vi "httpClient.vi"(8 "error in":errorcluster, 10 "data":string, 11 "URI":string) -> (0 "error out":errorcluster, 2 "code create":bool, 3 "HTTP Response Code":i32)   [LabVIEW 2015]
uses:
  <vilib>/httpClient/LabVIEWHTTPClient.lvlib
  <vilib>/Easy HTTP Client/HTTP Header.ctl
panel:
  out "headers":T1[](array[typedef])
  out "body":string
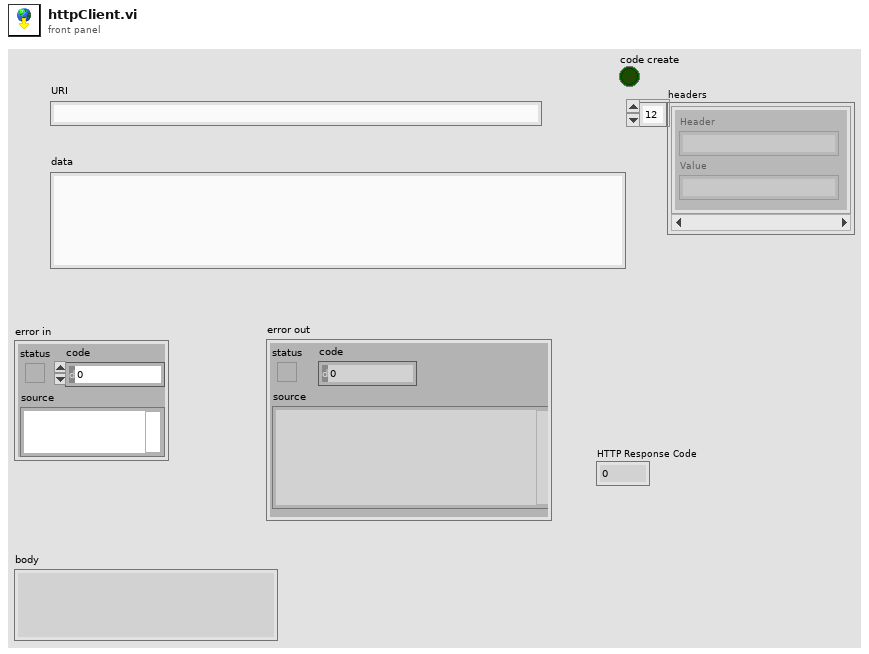
[diagram p1: front panel]
types:
  T1 = typedef "Easy HTTP.lvlib/HTTP Header.ctl" = cluster{"Header":string, "Value":string}
  T2 = typedef "LabVIEWHTTPClient.lvlib/ClientHandle.ctl" = refnum<k1>
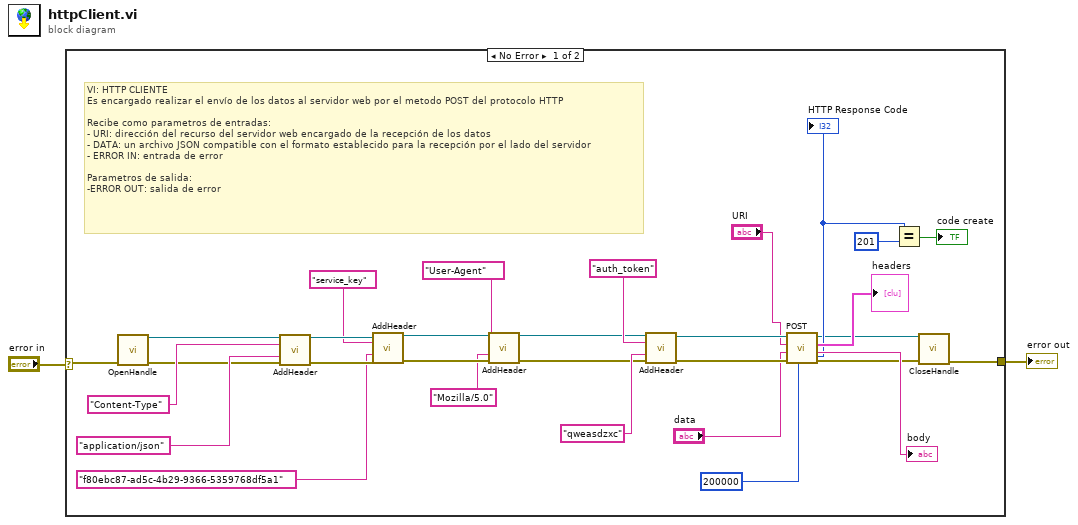
[diagram p0: block diagram]
diagram:
  n1 = case shown="No Error" "error in" {
    selector: "error in" -> [w6 w33]
    tunnel: [w4 w33] -> w1
    frame No Error {
      # "VI: HTTP CLIENTE\nEs encargado realizar el envío de los datos al servidor web por el metodo POST del protocolo HTTP\n\nRecibe como parametros de entradas:\n- URI: dirección del recurso del servidor web encargado de la recepción de los datos\n- DATA: un archivo JSON compatible con el formato establecido para la recepción por el lado del servidor\n- ERROR IN: entrada de error\n \nParametros de salida:\n-ERROR OUT: salida de error"
      n2 = call <vilib>:"OpenHandle.vi"("error in (no error)"=w6) -> ("client handle out"=w32:T2, "error out"=w29:errorcluster)  [unwired: 13 in]
      n3 = call <vilib>:"AddHeader.vi"("client handle"=w32, "header"="Content-Type", "value"="application/json", "error in (no error)"=w29) -> ("client handle out"=w28:T2, "error out"=w27:errorcluster)  [unwired: 10 in]
      n4 = call <vilib>:"AddHeader.vi"("client handle"=w28, "header"="service_key", "value"="f80ebc87-ad5c-4b29-9366-5359768df5a1", "error in (no error)"=w27) -> ("client handle out"=w22:T2, "error out"=w20:errorcluster)  [unwired: 10 in]
      n5 = call <vilib>:"AddHeader.vi"("client handle"=w22, "header"="User-Agent", "value"="Mozilla/5.0", "error in (no error)"=w20) -> ("client handle out"=w21:T2, "error out"=w19:errorcluster)  [unwired: 10 in]
      n6 = call <vilib>:"AddHeader.vi"("client handle"=w21, "header"="auth_token", "value"="qweasdzxc", "error in (no error)"=w19) -> ("client handle out"=w15:T2, "error out"=w16:errorcluster)  [unwired: 10 in]
      n7 = call <vilib>:"POST.vi"("timeout (10000)"=200000, "error in (no error)"=w16, "data"="data", "url"="URI", "client handle"=w15) -> ("error out"=w7:errorcluster, "body"=→"body":string, "headers"=→"headers":T1[], "client handle out"=w8:T2, "HTTP Response Code"=w10:i32)  [unwired: 2 in]
      "HTTP Response Code" <- w10
      n8 = Equal?(x=w10, y=201) -> (x = y?=→"code create":bool)
      n9 = call <vilib>:"CloseHandle.vi"("client handle"=w8, "error in (no error)"=w7) -> ("error out"=w4:errorcluster)  [unwired: 13 in]
    }
    frame Error {
    }
  }
  "error out" <- w1
